vi "test_Basic Deployment.vi"(8 "error in (no error)":errorcluster, 11 "Scalar Channels Testing in":refnum<class "Scalar Channels Testing.lvclass">) -> (0 "error out":errorcluster, 2 "System Definition Information":T1, 3 "Scalar Channels Testing out":refnum<class "Scalar Channels Testing.lvclass">)   [LabVIEW 2019, in "Scalar Channels Testing.lvclass"]
uses:
  Scalar Channels Testing.lvclass
  C:/Users/dstavila/Desktop/NI VeriStand FPGA Addon Fork/Source/Tests/FPGA Addon Test Class/FPGA Addon Test Class.lvclass
  C:/Program Files (x86)/National Instruments/LabVIEW 2019/vi.lib/NI/NI VeriStand Development Tools/NI Veristand Test Utilities/VeriStandTestCase/VeriStandTestCase.lvclass
  niveristand-custom-device-testing-tools/VeriStandTestUtilities/SystemDefinitionInformation.ctl
  niveristand-custom-device-testing-tools/VeriStandTestUtilities/TargetInformation.ctl
  niveristand-custom-device-testing-tools/VeriStandTestUtilities/ChassisInformation.ctl
  FPGA Addon Test Class/FPGA Addon Test Class.lvclass/FPGA Addon Test Class.ctl
  FPGA Addon Test Class/FPGA Addon Test Class.lvclass
  niveristand-custom-device-testing-tools/VeriStandTestUtilities/VeriStandTestUtilities.lvlib
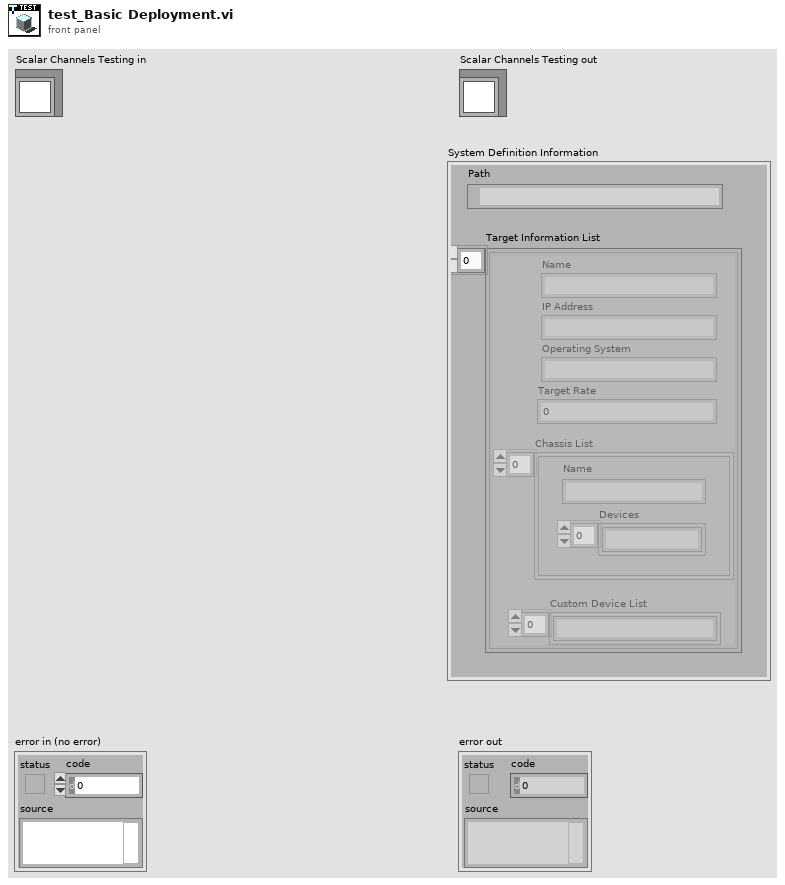
[diagram p1: front panel]
types:
  T1 = typedef "VeriStandTestUtilities.lvlib/SystemDefinitionInformation.ctl" = cluster{"Path":path, "Target Information List":T2[]}
  T2 = typedef "VeriStandTestUtilities.lvlib/TargetInformation.ctl" = cluster{"Name":string, "IP Address":string, "Operating System":string, "Target Rate":dbl, "Chassis List":T3[], "Custom Device List":string[]}
  T3 = typedef "VeriStandTestUtilities.lvlib/ChassisInformation.ctl" = cluster{"Name":string, "Devices":string[]}
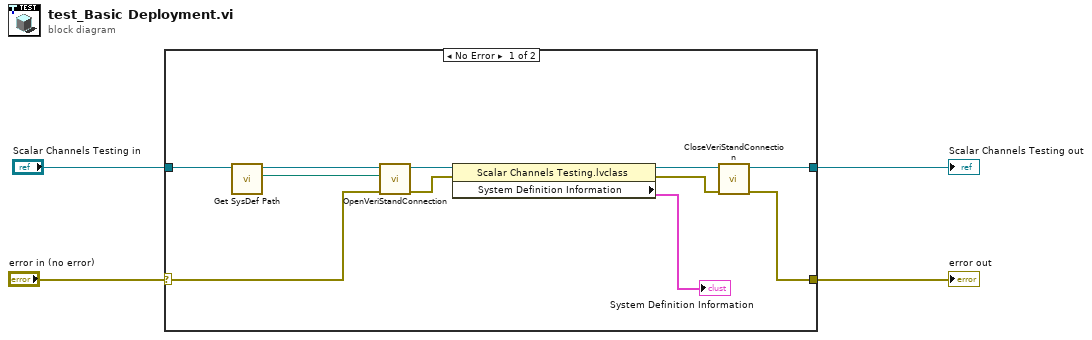
[diagram p0: block diagram]
diagram:
  n1 = case shown="No Error" "error in (no error)" {
    selector: "error in (no error)" -> [w10 w17]
    tunnel: [w9 w17] -> w4
    tunnel: [w11 w16] -> w2
    tunnel: "Scalar Channels Testing in" -> [w7 w16]
    frame No Error {
      n2 = call "Get SysDef Path.vi"("Scalar Channels Testing in"=w7) -> ("SysDef Path"=w5:path, "Scalar Channels Testing out"=w6:refnum<class "Scalar Channels Testing.lvclass">)  [unwired: 9 in]
      n3 = call-dynamic "OpenVeriStandConnection.vi"("error in (no error)"=w10, "System Definition File"=w5, "VeriStand Test Case in"=w6) -> ("error out"=w14:errorcluster, "VeriStand Test Case out"=w15:refnum<class "Scalar Channels Testing.lvclass">)  [unwired: 6 in, 1 out]
      n4 = property class="Scalar Channels Testing.lvclass"(reference=w15, error in=w14) -> (reference out=w13:refnum<class "Scalar Channels Testing.lvclass">, error out=w12:errorcluster, "System Definition Information"=→"System Definition Information":T1)
      n5 = call-dynamic "CloseVeriStandConnection.vi"("error in (no error)"=w12, "VeriStand Test Case in"=w13) -> ("error out"=w9:errorcluster, "VeriStand Test Case out"=w11:refnum<class "Scalar Channels Testing.lvclass">)  [unwired: 8 in]
    }
    frame Error {
    }
  }
  "error out" <- w4
  "Scalar Channels Testing out" <- w2
